vi "TestRedisData2Json.vi"() -> ()   [LabVIEW 2020]
panel:
  out "error out":errorcluster
  out "result string":string
  in  "data in":string
  out "JSON":string
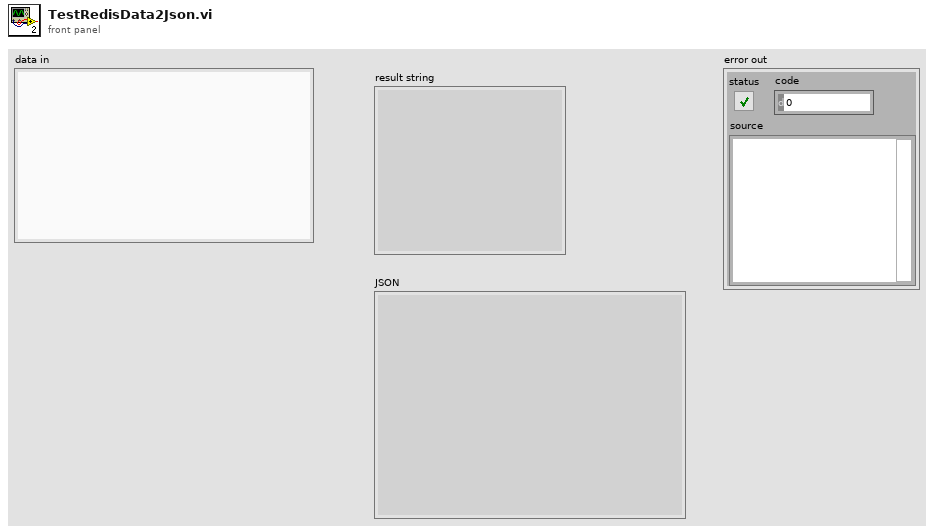
[diagram p1: front panel]
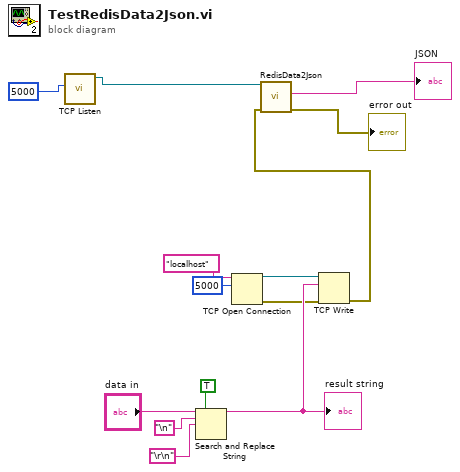
[diagram p0: block diagram]
diagram:
  n1 = call <vilib>:"TCP Listen.vi"("port"=u16 5000) -> ("connection ID"=w2:refnum<k5>)  [unwired: 6 in, 4 out]
  n2 = Search and Replace String(replace all?=TRUE ("replace all? (F)"), input string="data in", search string="\n", replace string="\r\n") -> (result string=w8:string)  [unwired: 4 in, 3 out]
  "result string" <- w8
  n3 = TCP Open Connection(address="localhost", remote port or service name=u16 5000) -> (connection ID=w5:refnum<k5>, error out=w4:errorcluster)  [unwired: 3 in]
  n4 = TCP Write(connection ID=w5, data in=w8, error in (no error)=w4) -> (error out=w13:errorcluster)  [unwired: 1 in, 2 out]
  n5 = call "RedisData2Json.vi"("error in"=w13, "RedisSession"=w2) -> ("error out"=→"error out":errorcluster, "JSON"=→"JSON":string)  [unwired: 6 in, 2 out]
